vi "SignalRead.vi"() -> ()   [LabVIEW 2012]
panel:
  in  "AddSpecial":bool
  in  "Remove":bool
  in  "Read":bool
  in  "Lista sygnałów":i32(listbox)
  out "Podgląd sygnału":dbl[](graph)
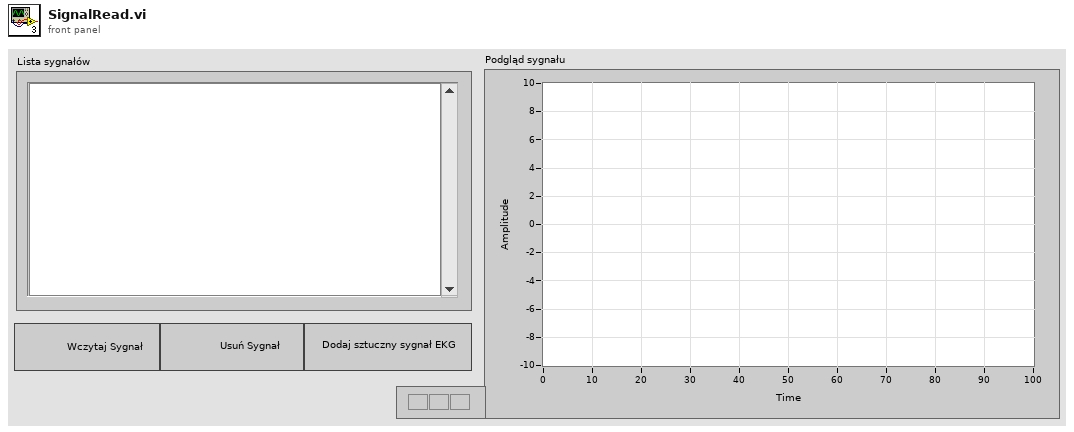
[diagram p1: front panel]
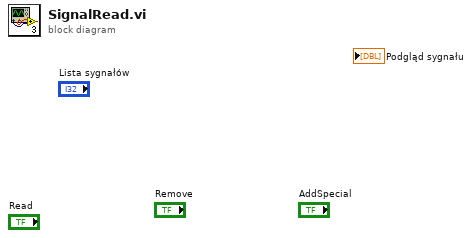
[diagram p0: block diagram]
diagram:
